vi "pixel_clock.vi"(7 "converter box version":i16=1 min=1 max=2, 10 "current iteration":u32, 11 "iterations per pixel":u32) -> ()   [LabVIEW 2010]
uses:
  <vilib>/eio/EIONode/EIONode.xnode
  <vilib>/rvi/eio/nirviEIOImplementation/nirviEIOImplementation.xnode
  <vilib>/rvi/eio/common/nirviEmuClasses.ctl
  <vilib>/rvi/eio/common/nirviEmuTemplateMethod_noerrors.vi
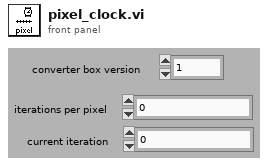
[diagram p1: front panel]
types:
  T1 = typedef "nirviEmuClasses.ctl" = enum16{"IO Read", "IO Write", "Method", "Property Read", "Property Write"}
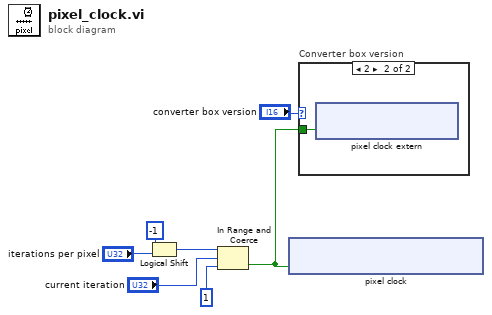
[diagram p0: block diagram]
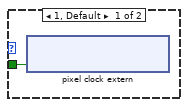
[diagram p2: hidden frame]
diagram:
  n1 = Logical Shift(y=i8 -1, x="iterations per pixel") -> (x << y=w7:u32)
  n2 = In Range and Coerce(upper limit=w7, x="current iteration", lower limit=u32 1 ("upper limit")) -> (In Range?=w2:bool)  [unwired: 1 out]
  n3 = xnode "pixel clock"("pixel clock (PCIe/PCIe_Trig3)"=w2) -> ()  [unwired: 1 in, 1 out]
  n4 = case "Converter box version" shown="2" "converter box version" {
    tunnel: w2 -> [w8 w20]
    frame 1, Default {
      n5 = xnode "pixel clock extern"("Connector1/DIO34"=w8) -> ()  [unwired: 1 in, 1 out]
    }
    frame 2 {
      n6 = xnode "pixel clock extern"("Connector2/DIO36"=w20) -> ()  [unwired: 1 in, 1 out]
    }
  }
